vi "Update FKs.vi"(8 "error in (no error)":errorcluster, 10 "Filter FK/PK":T1, 11 "Form Server in":refnum<class "Form Server.lvclass">) -> (0 "error out":errorcluster, 3 "Form Server out":refnum<class "Form Server.lvclass">)   [LabVIEW 2020, in "Form Server.lvlib" / "Form Server.lvclass"]
doc: "Determines which forms and fields to re-populate based registered FKs in the update fields logic object and the FK filter information. The FK filter information is specified by the update fields logic class."
uses:
  Form Server.lvclass
  Update Fields Logic/Field FK PK Info.ctl
  Form Server.lvclass/Form Server.ctl
  Form Server Configuration/Form Server Configuration.lvclass/Form Server Configuration.ctl
  Forms Model/Form Model Interfaces/Form Model Messages Messages/Populate Fields Msg/Populate Fields Msg.lvclass/Populate Fields Msg.ctl
  <vilib>/ActorFramework/Message Enqueuer/Message Enqueuer.lvclass/Message Enqueuer.ctl
  0f86da09-adc0-47a7-9d81-c6203699a2fe.vi
  <vilib>/ActorFramework/Message Enqueuer/Enqueue.vi
  Forms Model/Form Model Interfaces/Form Model Messages Messages/Populate Fields Msg/Populate Fields Msg.lvclass
  C:/Program Files (x86)/National Instruments/LabVIEW 2020/vi.lib/ActorFramework/Message/Message.lvclass
  <userlib>/_OpenG.lib/array/array.llb/Search 1D Array (Variant)__ogtk.vi
  <userlib>/_OpenG.lib/array/array.llb/Index 1D Array Elements (String)__ogtk.vi
  <vilib>/ActorFramework/Message Priority Queue/Priority Enqueue.vi
  Update Fields Logic/Update Fields Logic.lvclass
  Form Server Configuration/Form Server Configuration.lvclass
  Form Server Interfaces.lvlib
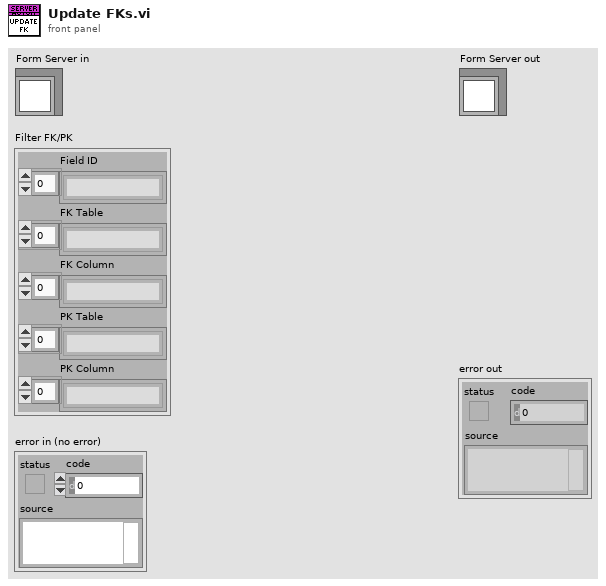
[diagram p1: front panel]
types:
  T1 = typedef "Form Server Interfaces.lvlib/Field FK PK Info.ctl" = cluster{"Field ID":string[], "FK Table":string[], "FK Column":string[], "PK Table":string[], "PK Column":string[]}
  T2 = typedef "Form Server Interfaces.lvlib/Form FK Fields.ctl" = cluster{"Form IDs":T3[], "Field IDs":string[]}
  T3 = typedef "Form Server Interfaces.lvlib/Form ID.ctl" = cluster{"Name":string, "Panel type":string}
  T4 = map{T3, refnum<class "Message Enqueuer.lvclass">}
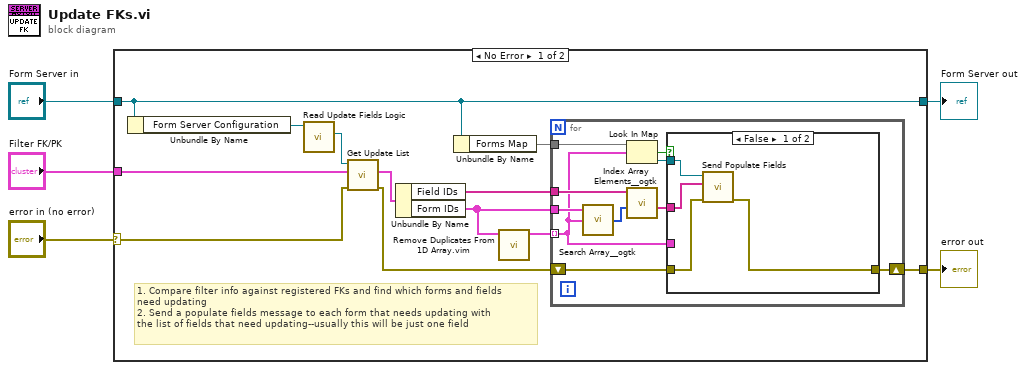
[diagram p0: block diagram]
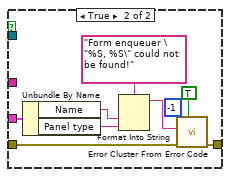
[diagram p2: hidden frame]
diagram:
  n1 = case shown="No Error" "error in (no error)" {
    selector: "error in (no error)" -> [w13 w42]
    tunnel: [w6 w42] -> w4
    tunnel: "Form Server in" -> [w12 w41]
    tunnel: [w12 w41] -> w2
    tunnel: "Filter FK/PK" -> [w15 _]
    frame No Error {
      # "1. Compare filter info against registered FKs and find which forms and fields\nneed updating\n2. Send a populate fields message to each form that needs updating with\nthe list of fields that need updating--usually this will be just one field"
      n2 = Unbundle By Name(w12) -> ("Form Server Configuration"=w17:refnum<class "Form Server Configuration.lvclass">)
      n3 = call "Read Update Fields Logic.vi"("Form Server Configuration in"=w17) -> ("Form Server Interfaces.lvlib:Update Fields Logic.lvclass"=w16:refnum<class "Update Fields Logic.lvclass">)  [unwired: 8 in, 2 out]
      n4 = call-dynamic "Get Update List.vi"("error in (no error)"=w13, "Filter FK/PK"=w15, "Update Fields Logic in"=w16) -> ("error out"=w7:errorcluster, "Fields to update"=w14:T2)  [unwired: 6 in, 1 out]
      n5 = Unbundle By Name(w14) -> ("Field IDs"=w9:string[], "Form IDs"=w10:T3[])
      n6 = Unbundle By Name(w12) -> ("Forms Map"=w8:T4)
      n7 = call "Remove Duplicates From 1D Array.vim"("array"=w10) -> ("array with duplicates removed"=w11:T3[])  [unwired: 10 in]
      n8 = for {
        tunnel: w11 -> [w18] mode=indexing
        tunnel: w10 -> [w27]
        tunnel: w9 -> [w25]
        tunnel: w8 -> [w24]
        shift-right: [w19] -> w6
        shift-left: w7 -> [w20]
        n9 = call-poly <userlib>:"Search Array__ogtk.vi"("Array"=w27, "Element Data"=w18) -> ("Indices of Elements"=w26:i32[])  [unwired: 7 in]
        n10 = Look In Map(map=w24, key=w18) -> (key not found?=w23:bool, value=w22:refnum<class "Message Enqueuer.lvclass">)  [unwired: 1 in]
        n11 = call-poly <userlib>:"Index Array Elements__ogtk.vi"("indices"=w26, "array"=w25) -> ("elements"=w21:string[])  [unwired: 9 in]
        n12 = case shown="False" w23 {
          tunnel: w22 -> [w31 _]
          tunnel: w21 -> [w30 _]
          tunnel: w20 -> [w29 w32]
          tunnel: [w28 w36] -> w19
          tunnel: w18 -> [_ w39]
          frame False {
            n13 = call "Send Populate Fields.vi"("error in (no error)"=w29, "Field Name Array (All)"=w30, "Message Enqueuer"=w31) -> ("error out"=w28:errorcluster)  [unwired: 7 in, 1 out]
          }
          frame True {
            n14 = Unbundle By Name(w39) -> ("Name"=w38:string, "Panel type"=w37:string)
            n15 = Format Into String(format string="Form enqueuer \"%S, %S\" could not be found!", w38, w37) -> (resulting string=w35:string)  [unwired: 2 in, 1 out]
            n16 = call <vilib>:"Error Cluster From Error Code.vi"("show call chain? (False)"=TRUE, "error in (no error)"=w32, "error message (\"\")"=w35, "error code (0)"=-1) -> ("error out"=w36:errorcluster)  [unwired: 5 in]
          }
        }
      }
    }
    frame Error {
    }
  }
  "error out" <- w4
  "Form Server out" <- w2
